vi "Read Rotation (incremental).vi"(8 "error in (no error)":errorcluster, 10 "reset":bool, 11 "Gyro bias":cluster{"X":dbl, "Y":dbl, "Z":dbl}) -> (0 "error out":errorcluster, 3 "Angle":cluster{"X":dbl, "Y":dbl, "Z":dbl}={"X"=0.0, "Y"=0.0, "Z"=1.5707963267948966})   [LabVIEW 2017]
uses:
  <vilib>/Analysis/coordinate.llb/Angle Range (Degree).ctl
  <vilib>/Analysis/coordinate.llb/Angle Units.ctl
  <vilib>/Analysis/coordinate.llb/Wrap Angle (scalar).vi
  Globals/Gyro.vi
  MPU6050 Read Rotation Data.vi
  Calculate Orientation.vi
  <vilib>/Analysis/NI_AAL_Angle.lvlib
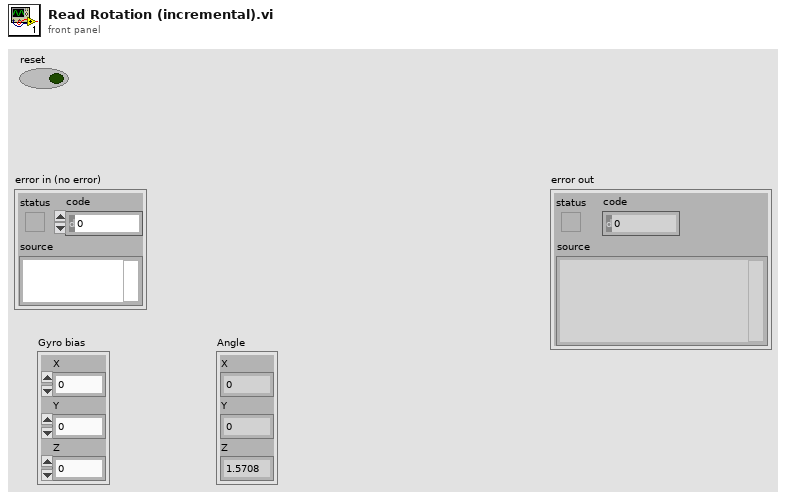
[diagram p1: front panel]
types:
  T1 = typedef "NI_AAL_Angle.lvlib/Angle Units.ctl" = i32
  T2 = typedef "NI_AAL_Angle.lvlib/Angle Range (Degree).ctl" = u16
  T3 = typedef "I2C.lvlib/I2C Reference.ctl" = cluster{"myRIO Reference":T4, "I2C Channels Enum":T8, "I2C Configuration":T9}
  T4 = typedef "myRIO Generic Hardware Reference.ctl" = cluster{"myRIO Model":T5, "myRIO Hardware Reference":T6}
  T5 = typedef "Hardware Version Enum.ctl" = enum16{"Unknown", "myRIO-1900", "myRIO-1950", "roboRIO", "NI ELVIS RIO CM"}
  T6 = typedef "myRIO v1.0 Reference.ctl" = cluster{"Generic FPGA Reference":T7, "Allow multiple opens":bool}
  T7 = typedef "Generic FPGA Reference.ctl" = refnum<k20>
  T8 = typedef "I2C Channels Enum.ctl" = enum16{"Not Connected", "A/I2C", "B/I2C", "I2C/I2C"}
  T9 = typedef "I2C.lvlib/I2C Configuration.ctl" = cluster{"I2C Transfer Rate":T10}
  T10 = typedef "I2C.lvlib/I2C Transfer Rate.ctl" = enum16{"Standard mode (100 kbps)", "Fast mode (400 kbps)"}
  T11 = cluster{"angle out":dbl, "angle out":dbl, "angle out":dbl}
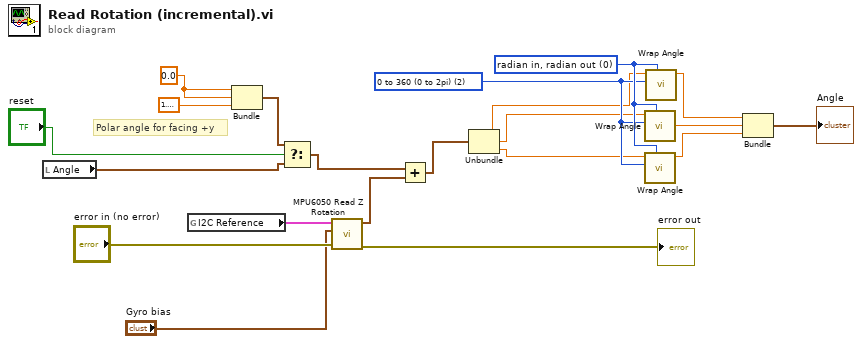
[diagram p0: block diagram]
diagram:
  w14 = 0.0
  w12 = T1 0 items=["radian in, radian out", "radian in, degree out", "degree in, degree out", "degree in, radian out"] ("angle units")
  w11 = T2 2 items=["none", "-180 to 180 (-pi to pi)", "0 to 360 (0 to 2pi)"] ("angle range")
  # "Polar angle for facing +y"
  n1 = local read "Angle"() -> (w18:cluster{"X":dbl, "Y":dbl, "Z":dbl})
  n2 = global read "Gyro.vi" "I2C Reference"() -> (w21:T3)
  n3 = Bundle(w14, w14, 1.5707963267948966) -> (w13:cluster{dbl, dbl, dbl})  [unwired: 1 in]
  n4 = Select(t=w13, s="reset", f=w18) -> (s? t:f=w17:cluster{"X":dbl, "Y":dbl, "Z":dbl})
  n5 = call "MPU6050 Read Z Rotation.vi"("error in (no error)"="error in (no error)", "Gyro bias"="Gyro bias", "I2C Ref In"=w21) -> ("error out"=→"error out":errorcluster, "Total Rotation (rads)"=w1:cluster{"X":dbl, "Y":dbl, "Z":dbl})  [unwired: 7 in]
  n6 = Add(x=w17, y=w1) -> (x+y=w10:cluster{"X":dbl, "Y":dbl, "Z":dbl})
  n7 = Unbundle(w10) -> ("X"=w3:dbl, "Y"=w4:dbl, "Z"=w5:dbl)
  n8 = call-poly <vilib>:"Wrap Angle.vi"("angle units"=w12, "angle range"=w11, "angle in"=w4) -> ("angle out"=w8:dbl)  [unwired: 7 in, 1 out]
  n9 = call-poly <vilib>:"Wrap Angle.vi"("angle units"=w12, "angle range"=w11, "angle in"=w5) -> ("angle out"=w7:dbl)  [unwired: 7 in, 1 out]
  n10 = call-poly <vilib>:"Wrap Angle.vi"("angle units"=w12, "angle range"=w11, "angle in"=w3) -> ("angle out"=w9:dbl)  [unwired: 7 in, 1 out]
  n11 = Bundle("angle out"=w9, "angle out"=w8, "angle out"=w7) -> (→"Angle":T11)  [unwired: 1 in]
